vi "NIIE_Eraser.vi"(8 "Error":errorcluster, 9 "Point Out":T1, 10 "Radio Buttons":T9=enum."Ellipse", 11 "Data":T2={"Class"={"Ants"=refnum, "Layer"=refnum, "Templates"=refnum, "Icon"=refnum, "Glyph"=refnum, "Settings"=refnum, "Tools"=refnum}, "Ref"={"Add Layer"=refnum, "Remove Layer"=refnum, "Line Text"=[], "Body Text Spec"=refnum, "DNL_Font"=refnum, "glyph path str"=refnum, "templates path str"=refnum, "Arrow Up"=refnum, "Arrow Down"=refnum, "IE VI Ref"=refnum, "Glyphs tree"=refnum, "Templates tree"=refnum, "Layer Icon Text"=refnum, "Layer Template"=refnum, "Clipboard"=refnum, "BW icon in"=refnum, "Color icon in"=refnum, "Layer Clust"=refnum, "Body Text"=refnum, "DNL_Framework Templates"=refnum, "Search Templates"=refnum, "TextMarker"=refnum, "Tab Control"=refnum, "Search Glyphs"=refnum, "Line Color"=refnum, "DNL_Glyphs []"=refnum, "Fill Color"=refnum, "Tools"=refnum, "Glyphs tree"=refnum, "Icon"=refnum, "Preview"=refnum, "Ants"=refnum, "Terminals"=refnum, "menu reference"=refnum, "LayerNames"=[], "GlyphLoadAnimation"=refnum, "TemplateLoadAnimation"=refnum, "refreshGlyphs"=refnum, "refreshTemplates"=refnum}, "Support"={"AntsRect"={"left"=0, "top"=0, "right"=0, "bottom"=0}, "Mouse Move Coords"={"Horizontal"=0, "Vertical"=0}, "Mouse Down Coords"={"Horizontal"=0, "Vertical"=0}, "Temp Coord"={"Horizontal"=0, "Vertical"=0}, "Action"=enum."Default", "Edge Color"=4914962, "Fill Color"=16860, "Mouse Down?"=FALSE, "Draft Mode?"=FALSE, "Temp Icon"=bytes[3102], "CTRL Pressed"=FALSE, "Move Selection?"=FALSE, "AntsRect Orig"={"left"=0, "top"=0, "right"=0, "bottom"=0}, "Text"="", "TM Set?"=FALSE, "Mouse inside icon?"=FALSE, "Tool (old value)"=0, "Pencil Move Color"=0, "Swap Colors?"=FALSE, "Shift pressed?"=FALSE}}) -> (0 "Error Out":errorcluster, 3 "Data Out":T2={"Class"={"Ants"=refnum, "Layer"=refnum, "Templates"=refnum, "Icon"=refnum, "Glyph"=refnum, "Settings"=refnum, "Tools"=refnum}, "Ref"={"Add Layer"=refnum, "Remove Layer"=refnum, "Line Text"=[], "Body Text Spec"=refnum, "DNL_Font"=refnum, "glyph path str"=refnum, "templates path str"=refnum, "Arrow Up"=refnum, "Arrow Down"=refnum, "IE VI Ref"=refnum, "Glyphs tree"=refnum, "Templates tree"=refnum, "Layer Icon Text"=refnum, "Layer Template"=refnum, "Clipboard"=refnum, "BW icon in"=refnum, "Color icon in"=refnum, "Layer Clust"=refnum, "Body Text"=refnum, "DNL_Framework Templates"=refnum, "Search Templates"=refnum, "TextMarker"=refnum, "Tab Control"=refnum, "Search Glyphs"=refnum, "Line Color"=refnum, "DNL_Glyphs []"=refnum, "Fill Color"=refnum, "Tools"=refnum, "Glyphs tree"=refnum, "Icon"=refnum, "Preview"=refnum, "Ants"=refnum, "Terminals"=refnum, "menu reference"=refnum, "LayerNames"=[], "GlyphLoadAnimation"=refnum, "TemplateLoadAnimation"=refnum, "refreshGlyphs"=refnum, "refreshTemplates"=refnum}, "Support"={"AntsRect"={"left"=0, "top"=0, "right"=0, "bottom"=0}, "Mouse Move Coords"={"Horizontal"=0, "Vertical"=0}, "Mouse Down Coords"={"Horizontal"=0, "Vertical"=0}, "Temp Coord"={"Horizontal"=0, "Vertical"=0}, "Action"=enum."Default", "Edge Color"=4914962, "Fill Color"=16860, "Mouse Down?"=FALSE, "Draft Mode?"=FALSE, "Temp Icon"=bytes[3102], "CTRL Pressed"=FALSE, "Move Selection?"=FALSE, "AntsRect Orig"={"left"=0, "top"=0, "right"=0, "bottom"=0}, "Text"="", "TM Set?"=FALSE, "Mouse inside icon?"=FALSE, "Tool (old value)"=0, "Pencil Move Color"=0, "Swap Colors?"=FALSE, "Shift pressed?"=FALSE}})   [LabVIEW 2021]
uses:
  MB CORE/TypeDefs/Cluster_Button Draw Tools.ctl
  MB CORE/TypeDefs/Bool_Draw Tool.ctl
  MB CORE/TypeDefs/Bool_Line Tool.ctl
  MB CORE/TypeDefs/Bool_ColorExtractor Tool.ctl
  MB CORE/TypeDefs/Bool_Fill Tool.ctl
  MB CORE/TypeDefs/Bool_IERect Tool.ctl
  MB CORE/TypeDefs/Bool_FRect Tool.ctl
  MB CORE/TypeDefs/Bool_Circle Tool.ctl
  MB CORE/TypeDefs/Bool_FillCircle Tool.ctl
  MB CORE/TypeDefs/Bool_Eraser Tool.ctl
  MB CORE/TypeDefs/Bool_Text Tool.ctl
  MB CORE/TypeDefs/Bool_Selection Tool.ctl
  MB CORE/TypeDefs/Bool_Move Tool.ctl
  Controls/IE Data.ctl
  Class/Ants/Ants.lvclass
  Class/FakedArray/FakedArray.lvclass
  vi.lib/LabVIEW Icon API/lv_icon/Classes/Icon/Icon.lvclass
  Class/Icon Library/Glyph.lvclass
  Class/Settings/Settings.lvclass
  Class/Tools/Tools Paint.lvclass
  Controls/IE Classes.ctl
  Controls/References Cluster.ctl
  Controls/SupportClass.ctl
  <vilib>/Utility/miscctls.llb/LVPoint32TypeDef.ctl
  Controls/ENUM_SupportClass_Action.ctl
  vi.lib/LabVIEW Icon API/lv_icon/Controls/IEColor.ctl
  <vilib>/Utility/miscctls.llb/LVPositionTypeDef.ctl
  vi.lib/LabVIEW Icon API/lv_icon/Classes/Icon Framework/Icon Framework.lvclass
  C:/Users/Mark.Balla/Projects/LV IconEditor Group/labview-icon-editor/vi.lib/LabVIEW Icon API/lv_icon/Classes/Layer/Layer.lvclass
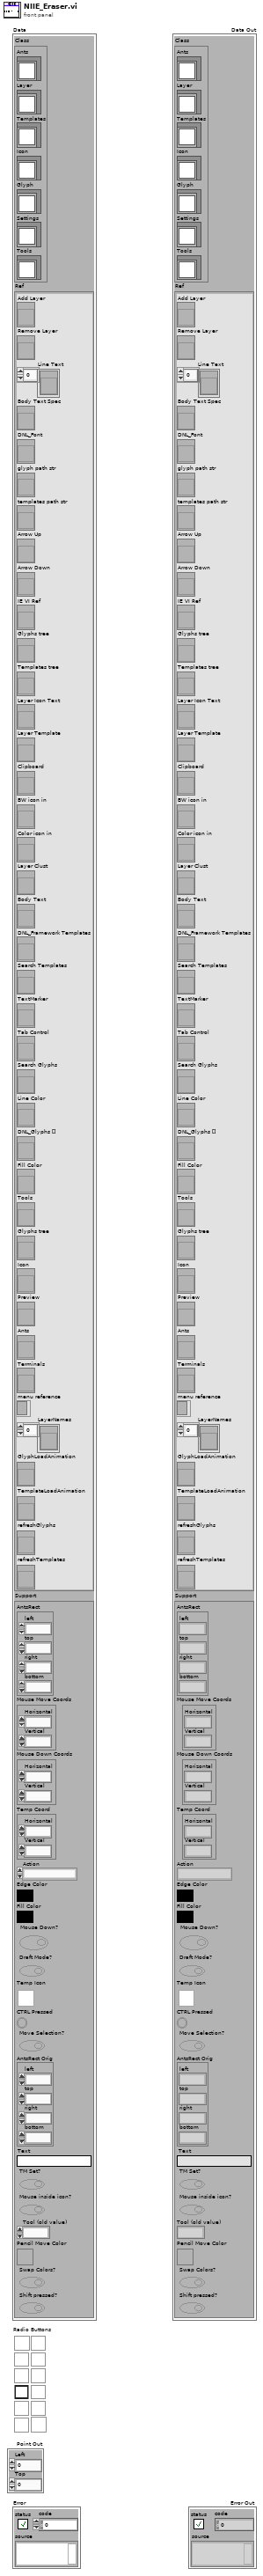
[diagram p1: front panel]
types:
  T1 = typedef "LVPositionTypeDef.ctl" = cluster{"Left":i32, "Top":i32}
  T2 = typedef "IE Data.ctl" = cluster{"Class":T3, "Ref":T4, "Support":T5}
  T3 = typedef "IE Classes.ctl" = cluster{"Ants":refnum<class "Ants.lvclass">, "Layer":refnum<class "FakedArray.lvclass">, "Templates":refnum<class "FakedArray.lvclass">, "Icon":refnum<class "Icon.lvclass">, "Glyph":refnum<class "Glyph.lvclass">, "Settings":refnum<class "Settings.lvclass">, "Tools":refnum<class "Tools Paint.lvclass">}
  T4 = typedef "References Cluster.ctl" = cluster{"Add Layer":refnum<vi>, "Remove Layer":refnum<vi>, "Line Text":refnum<vi>[], "Body Text Spec":refnum<vi>, "DNL_Font":refnum<vi>, "glyph path str":refnum<vi>, "templates path str":refnum<vi>, "Arrow Up":refnum<vi>, "Arrow Down":refnum<vi>, "IE VI Ref":refnum<vi>, "Glyphs tree":refnum<vi>, "Templates tree":refnum<vi>, "Layer Icon Text":refnum<vi>, "Layer Template":refnum<vi>, "Clipboard":refnum<vi>, "BW icon in":refnum<vi>, "Color icon in":refnum<vi>, "Layer Clust":refnum<vi>, "Body Text":refnum<vi>, "DNL_Framework Templates":refnum<vi>, "Search Templates":refnum<vi>, "TextMarker":refnum<vi>, "Tab Control":refnum<vi>, "Search Glyphs":refnum<vi>, "Line Color":refnum<vi>, "DNL_Glyphs []":refnum<vi>, "Fill Color":refnum<vi>, "Tools":refnum<vi>, "Glyphs tree":refnum<vi>, "Icon":refnum<vi>, "Preview":refnum<vi>, "Ants":refnum<vi>, "Terminals":refnum<vi>, "menu reference":refnum<k9>, "LayerNames":refnum<vi>[], "GlyphLoadAnimation":refnum<vi>, "TemplateLoadAnimation":refnum<vi>, "refreshGlyphs":refnum<vi>, "refreshTemplates":refnum<vi>}
  T5 = typedef "SupportClass.ctl" = cluster{"AntsRect":cluster{"left":i16, "top":i16, "right":i16, "bottom":i16}, "Mouse Move Coords":T6, "Mouse Down Coords":T6, "Temp Coord":T6, "Action":T7, "Edge Color":T8, "Fill Color":T8, "Mouse Down?":bool, "Draft Mode?":bool, "Temp Icon":picture, "CTRL Pressed":bool, "Move Selection?":bool, "AntsRect Orig":cluster{"left":i16, "top":i16, "right":i16, "bottom":i16}, "Text":string, "TM Set?":bool, "Mouse inside icon?":bool, "Tool (old value)":u32, "Pencil Move Color":u32, "Swap Colors?":bool, "Shift pressed?":bool}
  T6 = typedef "LVPoint32TypeDef.ctl" = cluster{"Horizontal":i32, "Vertical":i32}
  T7 = typedef "ENUM_SupportClass_Action.ctl" = enum16{"Default", "Move Selection", "Glyph Library", "Tool"}
  T8 = typedef "IEColor.ctl" = u32
  T9 = typedef "Cluster_Button Draw Tools.ctl" = enum32{"Pencil", "Line", "Dropper", "Fill", "Rectangle", "Filled Rectangle", "Ellipse", "Filled Ellipse", "Eraser", "Text", "Select", "Move"}
  T10 = typedef "Cluster_INI Data.ctl" = cluster{"Show Layer Tab?":bool, "Show Terminals?":bool, "Text":cluster{"Font":T11, "Alignment":T12, "Size":T13}, "3rd party Templates":cluster{"Store 3rd party Templates?":bool, "Folder Name":string}, "Merge user layers on commit":bool, "Body Text":T14, "Fill Color":T8, "Edge Color":T8, "Tab":u16, "Tool":T9, "Disable Layers?":bool}
  T11 = typedef "Font.ctl" = string
  T12 = typedef "Alignment.ctl" = u16
  T13 = typedef "Num_Font Size.ctl" = u8
  T14 = typedef "Cluster_BodyText.ctl" = cluster{"Line 1 text":string, "Line 2 text":string, "Line 3 text":string, "Line 4 text":string, "Line 1 color":u32, "Line 2 color":u32, "Line 3 color":u32, "Line 4 color":u32, "Body Text Spec":cluster{"Font":T11, "Alignment":T12, "Size":u8}, "Center text vertically":bool, "Capitalize Text":bool}
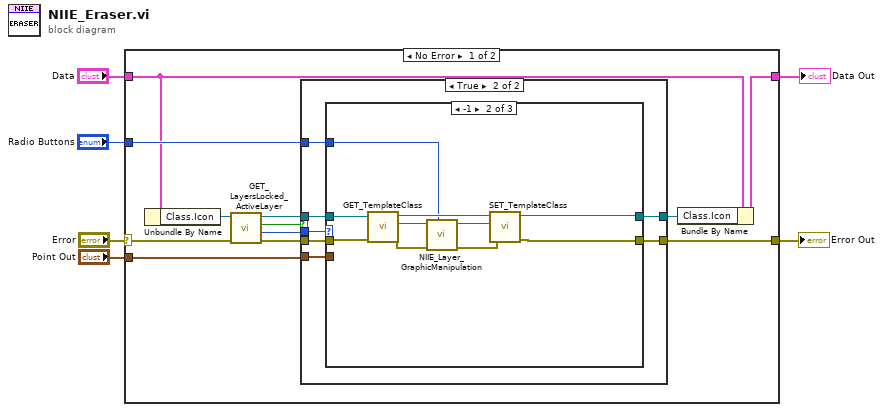
[diagram p0: block diagram]
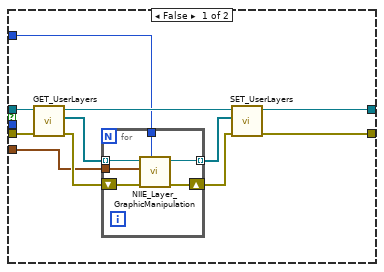
[diagram p2: hidden frame]
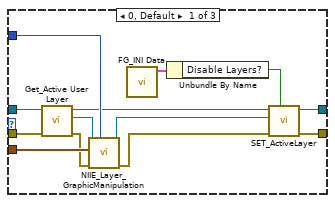
[diagram p3: hidden frame]
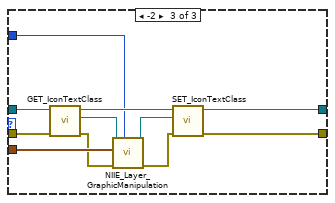
[diagram p4: hidden frame]
diagram:
  n1 = case shown="No Error" "Error" {
    selector: "Error" -> [w11 w78]
    tunnel: [w8 w78] -> w5
    tunnel: "Point Out" -> [w18 _]
    tunnel: "Radio Buttons" -> [w17 _]
    tunnel: "Data" -> [w10 w77]
    tunnel: [w7 w77] -> w2
    frame No Error {
      n2 = Unbundle By Name(w10) -> ("Class.Icon"=w12:refnum<class "Icon.lvclass">)
      n3 = call-dynamic "GET_LayersLocked_ActiveLayer.vi"("error in (no error)"=w11, "Icon.lvclass in"=w12) -> ("error out"=w15:errorcluster, "Active Layer"=w13:i32, "Layers Locked?"=w14:bool, "Icon.lvclass out"=w16:refnum<class "Icon.lvclass">)  [unwired: 6 out]
      n4 = case shown="True" w14 {
        tunnel: w18 -> [w24 w39]
        tunnel: w17 -> [w23 w38]
        tunnel: [w21 w37] -> w9
        tunnel: [w19 w36] -> w8
        tunnel: w16 -> [w22 w41]
        tunnel: w15 -> [w20 w40]
        tunnel: w13 -> [_ w42]
        frame False {
          n5 = call-dynamic "GET_UserLayers.vi"("error in (no error)"=w20, "Icon.lvclass in"=w22) -> ("error out"=w29:errorcluster, "All Layers"=w28:refnum<class "Layer.lvclass">[], "Icon.lvclass out"=w26:refnum<class "Icon.lvclass">)  [unwired: 7 out]
          n6 = for {
            tunnel: w28 -> [w34] mode=indexing
            tunnel: w24 -> [w35]
            tunnel: [w32] -> w27 mode=indexing
            shift-right: [w31] -> w25
            shift-left: w29 -> [w33]
            tunnel: w23 -> [w30]
            n7 = call "NIIE_Layer_GraphicManipulation.vi"("Radio Buttons"=w30, "Error"=w33, "Position"=w35, "Layer.lvclass"=w34) -> ("Error Out"=w31:errorcluster, "Layer.lvclass Out"=w32:refnum<class "Layer.lvclass">)  [unwired: 6 out]
          }
          n8 = call-dynamic "SET_UserLayers.vi"("error in (no error)"=w25, "Layers"=w27, "Icon.lvclass in"=w26) -> ("error out"=w19:errorcluster, "Icon.lvclass out"=w21:refnum<class "Icon.lvclass">)  [unwired: 7 out]
        }
        frame True {
          n9 = case shown="-1" w42 {
            tunnel: w41 -> [w55 w65 w76]
            tunnel: w40 -> [w54 w63 w75]
            tunnel: w39 -> [w52 _ w73]
            tunnel: w38 -> [w51 w56 w66]
            tunnel: [w48 w58 w68] -> w37
            tunnel: [w46 w57 w67] -> w36
            frame 0, Default {
              n10 = call-dynamic "Get_Active User Layer.vi"("error in (no error)"=w54, "Icon in"=w55) -> ("error out"=w49:errorcluster, "Layer.lvclass"=w53:refnum<class "Layer.lvclass">, "Icon out"=w50:refnum<class "Icon.lvclass">)  [unwired: 7 out]
              n11 = call "NIIE_Layer_GraphicManipulation.vi"("Radio Buttons"=w51, "Error"=w49, "Position"=w52, "Layer.lvclass"=w53) -> ("Error Out"=w47:errorcluster, "Layer.lvclass Out"=w45:refnum<class "Layer.lvclass">)  [unwired: 6 out]
              n12 = call "FG_INI Data.vi"() -> ("INI Data Out"=w44:T10)  [unwired: 1 in, 10 out]
              n13 = Unbundle By Name(w44) -> ("Disable Layers?"=w43:bool)
              n14 = call-dynamic "SET_ActiveLayer.vi"("Combine User Layers?"=w43, "Error"=w47, "Layer.lvclass"=w45, "Icon.lvclass"=w50) -> ("Error Out"=w46:errorcluster, "Icon.lvclass Out"=w48:refnum<class "Icon.lvclass">)  [unwired: 6 out]
            }
            frame -1 {
              n15 = call-dynamic "GET_TemplateClass.vi"("error in (no error)"=w63, "Icon.lvclass in"=w65) -> ("error out"=w62:errorcluster, "Icon Framework.lvclass"=w64:refnum<class "Icon Framework.lvclass">, "Icon.lvclass out"=w61:refnum<class "Icon.lvclass">)  [unwired: 7 out]
              n16 = call "NIIE_Layer_GraphicManipulation.vi"("Radio Buttons"=w56, "Error"=w62, "Layer.lvclass"=w64) -> ("Error Out"=w59:errorcluster, "Layer.lvclass Out"=w60:refnum<class "Icon Framework.lvclass">)  [unwired: 1 in, 6 out]
              n17 = call-dynamic "SET_TemplateClass.vi"("error in (no error)"=w59, "Icon Framework.lvclass"=w60, "Icon.lvclass in"=w61) -> ("error out"=w57:errorcluster, "Icon.lvclass out"=w58:refnum<class "Icon.lvclass">)  [unwired: 7 out]
            }
            frame -2 {
              n18 = call-dynamic "GET_IconTextClass.vi"("error in (no error)"=w75, "Icon.lvclass in"=w76) -> ("error out"=w72:errorcluster, "Icon Framework.lvclass"=w74:refnum<class "Icon Framework.lvclass">, "Icon.lvclass out"=w71:refnum<class "Icon.lvclass">)  [unwired: 7 out]
              n19 = call "NIIE_Layer_GraphicManipulation.vi"("Radio Buttons"=w66, "Error"=w72, "Position"=w73, "Layer.lvclass"=w74) -> ("Error Out"=w69:errorcluster, "Layer.lvclass Out"=w70:refnum<class "Icon Framework.lvclass">)  [unwired: 6 out]
              n20 = call-dynamic "SET_IconTextClass.vi"("error in (no error)"=w69, "Icon Framework.lvclass"=w70, "Icon.lvclass in"=w71) -> ("error out"=w67:errorcluster, "Icon.lvclass out"=w68:refnum<class "Icon.lvclass">)  [unwired: 7 out]
            }
          }
        }
      }
      n21 = Bundle By Name(cluster=w10, "Class.Icon"=w9) -> (w7:T2)
    }
    frame Error {
    }
  }
  "Error Out" <- w5
  "Data Out" <- w2
